vi "pathplan_vertices.vi"(0 "终点":dbl[](array[numeric]), 1 "车宽的一半":dbl=200.0, 2 "z_angle":dbl, 3 "起点":dbl[](array[numeric])) -> (7 "vertices":dbl[][](array[numeric]), 8 "distance_all":dbl, 9 "angle_all":dbl[](array[numeric]), 10 "distance_send_speed":dbl[](array[numeric]))   [LabVIEW 2016]
uses:
  <vilib>/imath/engines/lvmath2/RunTimeEngine/IndexRead/NIMS V(S).vi
  <instcachedir>/0/NIMS V(S)_0488751826AF41519A22953C041130DC.lvgen/NIMS V(S)_0488751826AF41519A22953C041130DC_000.vi
  <vilib>/imath/engines/lvmath2/RunTimeEngine/ErrorHandling/NIMS_Create Error From Enums.vi
  <vilib>/imath/engines/lvmath2/RunTimeEngine/BuiltInFunctions/length/NIMS_length(GV).vi
  <instcachedir>/0/NIMS_length(GV)_08A3D13377FD4E4B96F5795FBF3698FA.lvgen/NIMS_length(GV)_08A3D13377FD4E4B96F5795FBF3698FA_002.vi
  <vilib>/imathl/engines/lvmath/Functions/Error Handling/Create Error.vi
  <vilib>/imath/engines/lvmath/Functions/Error Handling/MergeErrorsWrapper.vi
  <vilib>/imath/engines/lvmath2/RunTimeEngine/VariableToken/NIMS_VariableToken_CondDefined.vi
  <instcachedir>/0/NIMS_VariableToken_CondDefined_06E9DA95BD4D46A6BA55EC651A891960.lvgen/NIMS_VariableToken_CondDefined_06E9DA95BD4D46A6BA55EC651A891960_003.vi
  <instcachedir>/0/NIMS_VariableToken_CondDefined_06E9DA95BD4D46A6BA55EC651A891960.lvgen/NIMS_VariableToken_CondDefined_06E9DA95BD4D46A6BA55EC651A891960_007.vi
  <vilib>/imath/engines/lvmath2/RunTimeEngine/BuiltInFunctions/size/NIMS_I32Row=size(GRow).vi
  <instcachedir>/0/NIMS_I32Row=size(GRow)_E5C05C6B13124B29B774CC4F993D3C59.lvgen/NIMS_I32Row=size(GRow)_E5C05C6B13124B29B774CC4F993D3C59_001.vi
  <vilib>/imath/engines/lvmath2/RunTimeEngine/IndexRead/NIMS M(S,S).vi
  <instcachedir>/0/NIMS M(S,S)_AC51E74150A542F7991B9634C66F3096.lvgen/NIMS M(S,S)_AC51E74150A542F7991B9634C66F3096_002.vi
  <vilib>/imath/engines/lvmath2/RunTimeEngine/IndexReplace/NIMS V(S)=S.vi
  <instcachedir>/0/NIMS V(S)=S_57E16554CB8B4B90AAB163894F717546.lvgen/NIMS V(S)=S_57E16554CB8B4B90AAB163894F717546_001.vi
  <instcachedir>/0/NIMS V(S)_0488751826AF41519A22953C041130DC.lvgen/NIMS V(S)_0488751826AF41519A22953C041130DC_003.vi
  <vilib>/imath/engines/lvmath2/RunTimeEngine/BuiltInFunctions/cos/NIMS_cos(C).vi
  <instcachedir>/0/NIMS_cos(C)_16E72F160CD540219ECD29F1B2AF26E5.lvgen/NIMS_cos(C)_16E72F160CD540219ECD29F1B2AF26E5_001.vi
  <vilib>/imath/engines/lvmath2/RunTimeEngine/BuiltInFunctions/abs/NIMS_abs(signed).vi
  <instcachedir>/0/NIMS_abs(signed)_C4FCB8E6058B49B797C7C8D53CA5F6EC.lvgen/NIMS_abs(signed)_C4FCB8E6058B49B797C7C8D53CA5F6EC_002.vi
  <vilib>/imath/engines/lvmath2/RunTimeEngine/RangeToken/NIMS_Range_R2 - Integer.vi
  <instcachedir>/0/NIMS_Range_R2 - Integer_89B873E74E6E489885E44F751DD9C6BF.lvgen/NIMS_Range_R2 - Integer_89B873E74E6E489885E44F751DD9C6BF_000.vi
  <vilib>/imath/engines/lvmath2/RunTimeEngine/CommandStatement/MC_CommandStatement_break.vi
  <instcachedir>/0/NIMS V(S)_0488751826AF41519A22953C041130DC.lvgen/NIMS V(S)_0488751826AF41519A22953C041130DC_002.vi
  <vilib>/imath/engines/lvmath2/RunTimeEngine/BuiltInFunctions/power/NIMS_power.vi
  <instcachedir>/0/NIMS_power_7E25183570944F38A5D8E4A9CE38EC54.lvgen/NIMS_power_7E25183570944F38A5D8E4A9CE38EC54_016.vi
  <instcachedir>/0/NIMS_abs(signed)_C4FCB8E6058B49B797C7C8D53CA5F6EC.lvgen/NIMS_abs(signed)_C4FCB8E6058B49B797C7C8D53CA5F6EC_000.vi
  <vilib>/imath/engines/lvmath2/RunTimeEngine/BuiltInFunctions/max/2 inputs/NIMS_max(RG,RG)-no size check.vi
  <instcachedir>/0/NIMS_max(RG,RG)-no size check_F871939977644B7683C1350DCCAD7557.lvgen/NIMS_max(RG,RG)-no size check_F871939977644B7683C1350DCCAD7557_000.vi
  <vilib>/imath/engines/lvmath2/RunTimeEngine/BuiltInFunctions/min/2 inputs/NIMS_min(RG,RG)-no size check.vi
  <instcachedir>/0/NIMS_min(RG,RG)-no size check_7F67BAB91AFC452D9517D2EA1C8F5F88.lvgen/NIMS_min(RG,RG)-no size check_7F67BAB91AFC452D9517D2EA1C8F5F88_001.vi
  <vilib>/imath/engines/lvmath2/RunTimeEngine/VariableToken/NIMS_VariableToken_CondDefinedDefinedByReplace.vi
  <instcachedir>/0/NIMS_VariableToken_CondDefinedDefinedByReplace_D162CFFC24174562A9FEA619A91E1A56.lvgen/NIMS_VariableToken_CondDefinedDefinedByReplace_D162CFFC24174562A9FEA619A91E1A56_002.vi
  <instcachedir>/0/NIMS V(S)=S_57E16554CB8B4B90AAB163894F717546.lvgen/NIMS V(S)=S_57E16554CB8B4B90AAB163894F717546_003.vi
  <vilib>/imath/engines/lvmath2/RunTimeEngine/ArithmeticOperatorToken/NIMS_ArithmeticOperator_minus.vi
  <instcachedir>/0/NIMS_ArithmeticOperator_minus_E3B65B1D26A44BB184AFDC5B3F458E3D.lvgen/NIMS_ArithmeticOperator_minus_E3B65B1D26A44BB184AFDC5B3F458E3D_003.vi
  <vilib>/imath/engines/lvmath2/RunTimeEngine/BuiltInFunctions/norm/NIMS_norm(GV,DBL).vi
  <instcachedir>/0/NIMS_norm(GV,DBL)_1268AFF3C646412B8C6EA3CE75D09042.lvgen/NIMS_norm(GV,DBL)_1268AFF3C646412B8C6EA3CE75D09042_000.vi
  <vilib>/imath/engines/lvmath2/RunTimeEngine/BuiltInFunctions/max/1 input/NIMS_max(RV).vi
  <instcachedir>/0/NIMS_max(RV)_237633DB1D604D5BA7001287DF3C7957.lvgen/NIMS_max(RV)_237633DB1D604D5BA7001287DF3C7957_002.vi
  <vilib>/imath/engines/lvmath2/RunTimeEngine/BuiltInFunctions/min/1 input/NIMS_min(RV).vi
  <instcachedir>/0/NIMS_min(RV)_EE2DD3E2888846108C5160A664B67832.lvgen/NIMS_min(RV)_EE2DD3E2888846108C5160A664B67832_002.vi
  <vilib>/imath/engines/lvmath2/RunTimeEngine/MatrixToken/NIMS_MatrixToken_RV_RV.vi
  <instcachedir>/0/NIMS_MatrixToken_RV_RV_41289AEE7DB340EFBB9CA44FA48DA89B.lvgen/NIMS_MatrixToken_RV_RV_41289AEE7DB340EFBB9CA44FA48DA89B_002.vi
  <vilib>/imath/engines/lvmath2/RunTimeEngine/MatrixToken/NIMS_MatrixToken_M_RV.vi
  <instcachedir>/0/NIMS_MatrixToken_M_RV_EE14907D4B194E829889005D2F556E9C.lvgen/NIMS_MatrixToken_M_RV_EE14907D4B194E829889005D2F556E9C_001.vi
  <vilib>/imath/engines/lvmath2/RunTimeEngine/IndexRead/NIMS V(V).vi
  <instcachedir>/0/NIMS V(V)_298D9CB7BFEB42B8BC8D9C3C28AE8C70.lvgen/NIMS V(V)_298D9CB7BFEB42B8BC8D9C3C28AE8C70_001.vi
  <vilib>/imath/engines/lvmath2/RunTimeSupport/NIMS_Get Scalar_w Error.vi
  <instcachedir>/0/NIMS_Get Scalar_w Error_59CA9FB130EE450F99234B5F2CCD930E.lvgen/NIMS_Get Scalar_w Error_59CA9FB130EE450F99234B5F2CCD930E_010.vi
  <instcachedir>/0/NIMS M(S,S)_AC51E74150A542F7991B9634C66F3096.lvgen/NIMS M(S,S)_AC51E74150A542F7991B9634C66F3096_000.vi
  <instcachedir>/0/NIMS_ArithmeticOperator_minus_E3B65B1D26A44BB184AFDC5B3F458E3D.lvgen/NIMS_ArithmeticOperator_minus_E3B65B1D26A44BB184AFDC5B3F458E3D_011.vi
  <vilib>/imath/engines/lvmath2/RunTimeEngine/IndexReplace/NIMS M($,S)=M.vi
  <instcachedir>/0/NIMS M($,S)=M_4ED09617E62F4BDFBC079C86D2836811.lvgen/NIMS M($,S)=M_4ED09617E62F4BDFBC079C86D2836811_000.vi
  <vilib>/imath/engines/lvmath2/RunTimeEngine/IndexReplace/NIMS M(S,S)=S.vi
  <instcachedir>/0/NIMS M(S,S)=S_98E40400474E4398B113AE20298B4F82.lvgen/NIMS M(S,S)=S_98E40400474E4398B113AE20298B4F82_000.vi
  <vilib>/imath/engines/lvmath2/RunTimeEngine/RowToken/NIMS_RowToken_CV_CV.vi
  <instcachedir>/0/NIMS_RowToken_CV_CV_5546A0B1CA2C4E49826F811B9C073FB0.lvgen/NIMS_RowToken_CV_CV_5546A0B1CA2C4E49826F811B9C073FB0_000.vi
  <vilib>/imath/engines/lvmath2/RunTimeEngine/IndexRead/NIMS M($,S).vi
  <instcachedir>/0/NIMS M($,S)_3E5749BBB62E49528D4765A77F1F6D98.lvgen/NIMS M($,S)_3E5749BBB62E49528D4765A77F1F6D98_002.vi
  <instcachedir>/0/NIMS_min(RG,RG)-no size check_7F67BAB91AFC452D9517D2EA1C8F5F88.lvgen/NIMS_min(RG,RG)-no size check_7F67BAB91AFC452D9517D2EA1C8F5F88_002.vi
  <instcachedir>/0/NIMS_max(RG,RG)-no size check_F871939977644B7683C1350DCCAD7557.lvgen/NIMS_max(RG,RG)-no size check_F871939977644B7683C1350DCCAD7557_001.vi
  <vilib>/imath/engines/lvmath2/RunTimeEngine/RowToken/NIMS_RowToken_M_CV.vi
  <instcachedir>/0/NIMS_RowToken_M_CV_FA79F1D1D17D44459F3ED8E09EE8B625.lvgen/NIMS_RowToken_M_CV_FA79F1D1D17D44459F3ED8E09EE8B625_000.vi
  <vilib>/imath/engines/lvmath2/RunTimeEngine/BuiltInFunctions/mirrorh/NIMS_mirrorh(GM).vi
  <instcachedir>/0/NIMS_mirrorh(GM)_A650AD0D730A4A8EBE251B4C5C7CA115.lvgen/NIMS_mirrorh(GM)_A650AD0D730A4A8EBE251B4C5C7CA115_005.vi
  <instcachedir>/0/NIMS M($,S)_3E5749BBB62E49528D4765A77F1F6D98.lvgen/NIMS M($,S)_3E5749BBB62E49528D4765A77F1F6D98_000.vi
  <vilib>/imath/engines/lvmath2/RunTimeEngine/RelationalOperatorToken/NIMS_Relational_Operator_Eq.vi
  <instcachedir>/0/NIMS_Relational_Operator_Eq_FD198F059617437A8A02361002FCA645.lvgen/NIMS_Relational_Operator_Eq_FD198F059617437A8A02361002FCA645_006.vi
  <vilib>/imath/engines/lvmath2/RunTimeEngine/IndexRead/NIMS M($,R2).vi
  <instcachedir>/0/NIMS M($,R2)_D9380E19261A4ADFB2D364AF6959C6EF.lvgen/NIMS M($,R2)_D9380E19261A4ADFB2D364AF6959C6EF_001.vi
  <vilib>/imath/engines/lvmath2/RunTimeEngine/RowToken/NIMS_RowToken_M_M.vi
  <instcachedir>/0/NIMS_RowToken_M_M_968CDE3545E74ACDAEA4B48DE01EEECA.lvgen/NIMS_RowToken_M_M_968CDE3545E74ACDAEA4B48DE01EEECA_004.vi
  <vilib>/imath/engines/lvmath2/RunTimeEngine/BuiltInFunctions/length/NIMS_length(GM).vi
  <instcachedir>/0/NIMS_length(GM)_47CEC356FCE0482D9BA47DC61C99F2C7.lvgen/NIMS_length(GM)_47CEC356FCE0482D9BA47DC61C99F2C7_000.vi
  <vilib>/imath/engines/lvmath2/RunTimeEngine/BuiltInFunctions/dot/NIMS_dot(GV,GV).vi
  <instcachedir>/0/NIMS_dot(GV,GV)_B9FAA411F4494E9B94D442721014A3FA.lvgen/NIMS_dot(GV,GV)_B9FAA411F4494E9B94D442721014A3FA_000.vi
  <vilib>/imath/engines/lvmath2/RunTimeEngine/RowToken/NIMS_RowToken_M_SorRV.vi
  <instcachedir>/0/NIMS_RowToken_M_SorRV_4D710C5E6F8040F3A39B2F03436798DB.lvgen/NIMS_RowToken_M_SorRV_4D710C5E6F8040F3A39B2F03436798DB_002.vi
  <instcachedir>/0/NIMS_abs(signed)_C4FCB8E6058B49B797C7C8D53CA5F6EC.lvgen/NIMS_abs(signed)_C4FCB8E6058B49B797C7C8D53CA5F6EC_005.vi
  <vilib>/imath/engines/lvmath2/RunTimeEngine/VariableToken/Support/NIMS_Matrix Boolean Index to I32 Index.vi
  <vilib>/imath/engines/lvmath2/RunTimeEngine/IndexReplace/NIMS M(V)=S.vi
  <instcachedir>/0/NIMS M(V)=S_F2304187E1344F60ABCBE5C5CC0920F9.lvgen/NIMS M(V)=S_F2304187E1344F60ABCBE5C5CC0920F9_000.vi
  <vilib>/imath/engines/lvmath2/RunTimeEngine/BuiltInFunctions/size/NIMS_I32=size(GM,I32).vi
  <instcachedir>/0/NIMS_I32=size(GM,I32)_122058B1B3294FAEA5DC209B92B394E4.lvgen/NIMS_I32=size(GM,I32)_122058B1B3294FAEA5DC209B92B394E4_004.vi
  <instcachedir>/0/NIMS_RowToken_M_SorRV_4D710C5E6F8040F3A39B2F03436798DB.lvgen/NIMS_RowToken_M_SorRV_4D710C5E6F8040F3A39B2F03436798DB_003.vi
  <vilib>/imath/engines/lvmath2/RunTimeEngine/IndexRead/NIMS M(S).vi
  <instcachedir>/0/NIMS M(S)_B826C018497E4940AE96BD27B540B6FB.lvgen/NIMS M(S)_B826C018497E4940AE96BD27B540B6FB_000.vi
  <vilib>/imath/engines/lvmath2/RunTimeEngine/IndexReplace/NIMS M($,S)=V.vi
  <instcachedir>/0/NIMS M($,S)=V_EEA74323A7E5479BB387BE0F93352290.lvgen/NIMS M($,S)=V_EEA74323A7E5479BB387BE0F93352290_001.vi
  <vilib>/imath/engines/lvmath2/RunTimeEngine/RowToken/NIMS_RowToken_SorRV_M.vi
  <instcachedir>/0/NIMS_RowToken_SorRV_M_1F580C56DFC142B492C663A3FF978087.lvgen/NIMS_RowToken_SorRV_M_1F580C56DFC142B492C663A3FF978087_000.vi
  <vilib>/imath/engines/lvmath2/RunTimeEngine/NodeEndStatement/NIMS_NodeEndStatement_Get Vector.vi
  <instcachedir>/0/NIMS_NodeEndStatement_Get Vector_9E4547DF38A84F62A7E036B4CE3D251C.lvgen/NIMS_NodeEndStatement_Get Vector_9E4547DF38A84F62A7E036B4CE3D251C_001.vi
  <vilib>/imath/engines/lvmath2/RunTimeEngine/NodeEndStatement/NIMS_NodeEndStatement_Output.vi
  <instcachedir>/0/NIMS_NodeEndStatement_Output_53EC0D466D134D7ABD903AC30B43404B.lvgen/NIMS_NodeEndStatement_Output_53EC0D466D134D7ABD903AC30B43404B_005.vi
  <instcachedir>/0/NIMS_NodeEndStatement_Output_53EC0D466D134D7ABD903AC30B43404B.lvgen/NIMS_NodeEndStatement_Output_53EC0D466D134D7ABD903AC30B43404B_002.vi
  <instcachedir>/0/NIMS_NodeEndStatement_Output_53EC0D466D134D7ABD903AC30B43404B.lvgen/NIMS_NodeEndStatement_Output_53EC0D466D134D7ABD903AC30B43404B_001.vi
  <vilib>/imath/engines/lvmath2/RunTimeEngine/ErrorHandling/NIMS_Finalize Error.vi
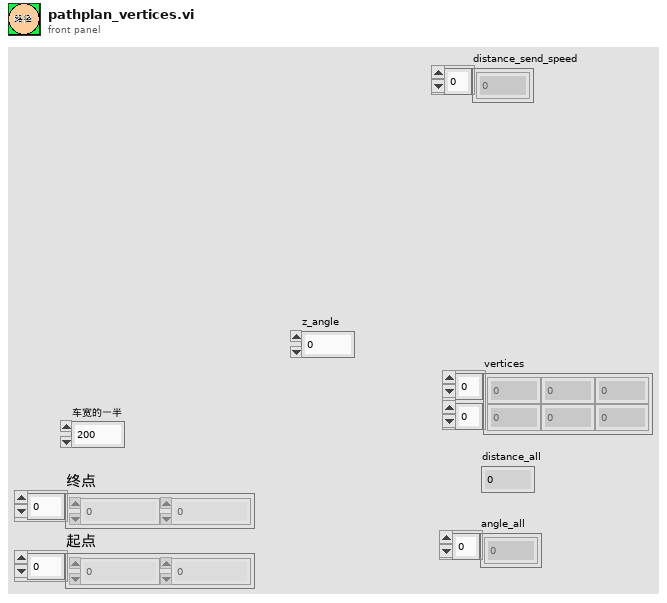
[diagram p1: front panel]
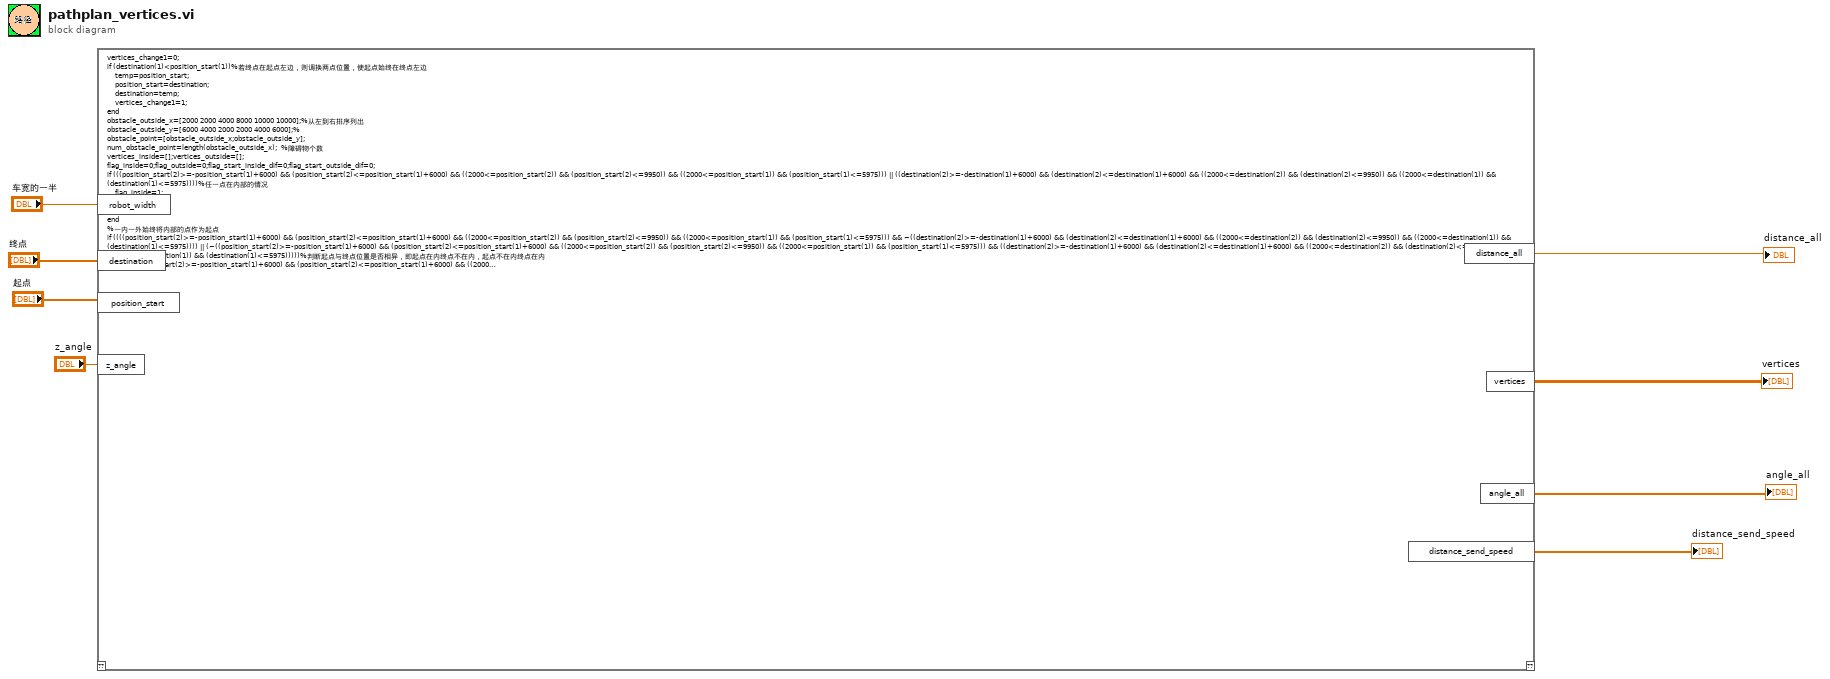
[diagram p0: block diagram]
diagram:
  n1 = mathscript code="vertices_change1=0;\nif (destination(1)<position_start(1))%若终点在起点左边，则调换两点位置，使起点始终在终点左边\n    temp=position_start;\n    position_start=destination;\n    destination=temp;\n    vertices_change1=1;\nend\nobstacle_outside_x=[2000 2000 4000 8000 10000 10000];%从左到右排序列出\nobstacle_outside_y=[6000 4000 2000 2000 4000 6000];%\nobstacle_point=[obstacle_outside_x;obstacle_outside_y];  \nnum_obstacle_point=length(obstacle_outside_x);  %障碍物个数\nvertices_inside=[];vertices_outside=[];\nflag_inside=0;flag_outside=0;flag_start_inside_dif=0;flag_start_outside_dif=0;\nif (((position_start(2)>=-position_start(1)+6000) && (position_start(2)<=position_start(1)+6000) && ((2000<=position_start(2)) && (position_start(2)<=9950)) && ((2000<=position_start(1)) && (position_start(1)<=5975))) || ((destination(2)>=-destination(1)+6000) && (destination(2)<=destination(1)+6000) && ((2000<=destination(2)) && (destination(2)<=9950)) && ((2000<=destination(1)) && (destination(1)<=5975))))%任一点在内部的情况\n    flag_inside=1;\nelse\n    flag_outside=1;\nend\n%一内一外始终将内部的点作为起点\nif ((((position_start(2)>=-position_start(1)+6000) && (position_start(2)<=position_start(1)+6000) && ((2000<=position_start(2)) && (position_start(2)<=9950)) && ((2000<=position_start(1)) && (position_start(1)<=5975))) && ~((destination(2)>=-destination(1)+6000) && (destination(2)<=destination(1)+6000) && ((2000<=destination(2)) && (destination(2)<=9950)) && ((2000<=destination(1)) && (destination(1)<=5975)))) || (~((position_start(2)>=-position_start(1)+6000) && (position_start(2)<=position_start(1)+6000) && ((2000<=position_start(2)) && (position_start(2)<=9950)) && ((2000<=position_start(1)) && (position_start(1)<=5975))) && ((destination(2)>=-destination(1)+6000) && (destination(2)<=destination(1)+6000) && ((2000<=destination(2)) && (destination(2)<=9950)) && ((2000<=destination(1)) && (destination(1)<=5975)))))%判断起点与终点位置是否相异，即起点在内终点不在内，起点不在内终点在内\n    if ((position_start(2)>=-position_start(1)+6000) && (position_start(2)<=position_start(1)+6000) && ((2000<=position_start(2)) && (position_start(2)<=9950)) && ((2000<=position_start(1)) && (position_start(1)<=5975)))%起点在内，终点在外\n        flag_start_inside_dif=1;%标记相异\n    else\n        flag_start_outside_dif=1;%标记相异，起点在外面，将点交换，内部的点作为起点\n        temp=position_start;\n        position_start=destination;\n        destination=temp;\n    end \n    position_start_inside=position_start;\n    destination_in2out=[5700 1750];%从内部到外部的目标点\nend\n\nif (flag_inside || flag_start_inside_dif || flag_start_outside_dif)%点在内部的情况\n    if (flag_start_inside_dif || flag_start_outside_dif) %如果内外相异\n        position_destination_inside=destination_in2out;\n    else   %内外不相异\n        position_start_inside=position_start;\n        position_destination_inside=destination;\n    end      \n    vertices_inside=[position_start_inside]';\n    obstacle_inside_x=[4000 6000 6000 6000];%\n    obstacle_inside_y=[6000 3500 6000 8500];%\n    size_obstacle=size(obstacle_inside_x);        %障碍物个数\n    num_obstacle=size_obstacle(1,2);\n    count=0;\n    x=[];y=[];\n    radius=150+100;\n    beta(1)=atan((position_start_inside(2)-position_destination_inside(2))/(position_start_inside(1)-position_destination_inside(1)));\n    robot_dis_obs=abs((robot_width+radius)/cos(beta(1)));\n    k=(position_start_inside(2)-position_destination_inside(2))/(position_start_inside(1)-position_destination_inside(1));\n    b=k*(-position_start_inside(1))+position_start_inside(2);\n    flag=0;\n    %判断直行路径范围内是否有障碍物，如果有记录障碍物点做标\n    if num_obstacle==0\n        x=[position_start_inside(1),position_destination_inside(1)];\n        y=[position_start_inside(2),position_destination_inside(2)];\n    else\n    for i=1:num_obstacle\n        line_k=k;line_b=b;array_o=[obstacle_inside_x(i),obstacle_inside_y(i)];\n        if line_k==inf||line_k==-inf\n            dis_dot_line=abs(array_o(2)-line_b);\n        else\n            molecule=(line_k*array_o(1)-array_o(2)+line_b);\n            dis_dot_line=abs(molecule/sqrt(power(line_k,2)+1));\n        end\n        dis_line=dis_dot_line;\n        if (dis_line<robot_width+radius || dis_line==robot_width+radius)&&(obstacle_inside_x(i)<max(position_destination_inside(1),position_start_inside(1))+robot_width+radius&&obstacle_inside_x(i)>min(position_destination_inside(1),position_start_inside(1))-robot_width+radius&&obstacle_inside_y(i)<max(position_destination_inside(2),position_start_inside(2))+robot_width+radius&&obstacle_inside_y(i)>min(position_destination_inside(2),position_start_inside(2))-robot_width+radius)\n            in_obstacle(count+1)=obstacle_inside_x(i);\n            in_obstacle(count+2)=obstacle_inside_y(i);\n            count=count+2;\n        end\n    end\n    cosalph=(position_start_inside(1)-position_destination_inside(1))/norm(position_destination_inside-position_start_inside);\n    sinalph=(position_start_inside(2)-position_destination_inside(2))/norm(position_destination_inside-position_start_inside);\n    if position_start_inside(1)<position_destination_inside(1)\n        cosalph=-cosalph;\n        sinalph=-sinalph;\n    end\n        if (count==0)       %(k==inf||k==-inf)||\n            x=[position_start_inside(1),position_destination_inside(1)];\n            y=[position_start_inside(2),position_destination_inside(2)];\n            vertices_inside=[vertices_inside,position_destination_inside'];\n        else\n            %关于障碍物点x、y轴的偏移量\n            x_offset=(robot_width+radius);\n            y_offset=(robot_width+radius);\n            %旋转坐标系下的偏移量\n            a_cos=x_offset*cosalph;a_sin=x_offset*sinalph;\n            b_cos=y_offset*cosalph;b_sin=y_offset*sinalph;\n\n            if count==2 %一个障碍物\n                %当障碍物在两点连线上方时\n                if (in_obstacle(2)>(k*in_obstacle(1)+b))||(k==inf&&position_destination_inside(1)>obstacle_inside_x(i))\n                    %先进行选取四点坐标\n                    temp_position1=[in_obstacle(1)+a_cos+b_sin,in_obstacle(2)+a_sin-b_cos];\n                    temp_position2=[in_obstacle(1)-a_cos+b_sin,in_obstacle(2)-a_sin-b_cos];\n                    if position_start_inside(1)>position_destination_inside(1)\n                        if temp_position1(1)>temp_position2(1)\n                            vertices_inside=[position_start_inside;temp_position1;temp_position2;position_destination_inside]';\n                        else\n                            vertices_inside=[position_start_inside;temp_position2;temp_position1;position_destination_inside]';\n                        end\n                    else\n                        if temp_position1(1)>temp_position2(1)\n                            vertices_inside=[position_start_inside;temp_position2;temp_position1;position_destination_inside]';\n                        else\n                            vertices_inside=[position_start_inside;temp_position1;temp_position2;position_destination_inside]';\n                        end\n                    end\n                else\n                    temp_position1=[in_obstacle(1)+a_cos-b_sin,in_obstacle(2)+a_sin+b_cos];\n                    temp_position2=[in_obstacle(1)-a_cos-b_sin,in_obstacle(2)-a_sin+b_cos];\n                    if position_start_inside(1)>position_destination_inside(1)\n                        if temp_position1(1)>temp_position2(1)\n                            vertices_inside=[position_start_inside;temp_position1;temp_position2;position_destination_inside]';\n                        else\n                            vertices_inside=[position_start_inside;temp_position2;temp_position1;position_destination_inside]';\n                        end\n                    else\n                        if temp_position1(1)>temp_position2(1)\n                            vertices_inside=[position_start_inside;temp_position2;temp_position1;position_destination_inside]';\n                        else\n                            vertices_inside=[position_start_inside;temp_position1;temp_position2;position_destination_inside]';\n                        end\n                    end\n                    for i=1:num_obstacle\n                         if (obstacle_inside_x(i)~=in_obstacle(1))&&(obstacle_inside_x(i)<max(vertices_inside(1,1),vertices_inside(1,2))&&obstacle_inside_x(i)>min(vertices_inside(1,1),vertices_inside(1,2)))&&(obstacle_inside_y(i)<((vertices_inside(2,2)-vertices_inside(2,1))/(vertices_inside(1,2)-vertices_inside(1,1))*obstacle_inside_x(i)+vertices_inside(2,2)-(vertices_inside(2,2)-vertices_inside(2,1))/(vertices_inside(1,2)-vertices_inside(1,1))*vertices_inside(1,2)+robot_dis_obs))&&(obstacle_inside_y(i)>((vertices_inside(2,2)-vertices_inside(2,1))/(vertices_inside(1,2)-vertices_inside(1,1))*obstacle_inside_x(i)+vertices_inside(2,2)-(vertices_inside(2,2)-vertices_inside(2,1))/(vertices_inside(1,2)-vertices_inside(1,1))*vertices_inside(1,2)-robot_dis_obs))||(obstacle_inside_x(i)~=in_obstacle(1))&&(obstacle_inside_x(i)<max(vertices_inside(1,3),vertices_inside(1,4))&&obstacle_inside_x(i)>min(vertices_inside(1,3),vertices_inside(1,4)))&&(obstacle_inside_y(i)<((vertices_inside(2,4)-vertices_inside(2,3))/(vertices_inside(1,4)-vertices_inside(1,3))*obstacle_inside_x(i)+vertices_inside(2,4)-(vertices_inside(2,4)-vertices_inside(2,3))/(vertices_inside(1,4)-vertices_inside(1,3))*vertices_inside(1,4)+robot_dis_obs))&&(obstacle_inside_y(i)>((vertices_inside(2,4)-vertices_inside(2,3))/(vertices_inside(1,4)-vertices_inside(1,3))*obstacle_inside_x(i)+vertices_inside(2,4)-(vertices_inside(2,4)-vertices_inside(2,3))/(vertices_inside(1,4)-vertices_inside(1,3))*vertices_inside(1,4)-robot_dis_obs))\n                            in_obstacle(count+1)=obstacle_inside_x(i);\n                            in_obstacle(count+2)=obstacle_inside_y(i);\n                            count=count+2;\n                            break;\n                        end\n                    end\n                end\n            else\n                if k*max(obstacle_inside_x)+b<min(obstacle_inside_y)\n                    temp_position1=[max(obstacle_inside_x)+x_offset,min(obstacle_inside_y)+y_offset];\n                    temp_position2=[max(obstacle_inside_x)-x_offset,min(obstacle_inside_y)+y_offset];\n                    if norm(position_start_inside-temp_position1)<norm(position_start_inside-temp_position2)\n                        temp1=temp_position1;\n                        temp2=temp_position2;\n                    else\n                        temp1=temp_position2;\n                        temp2=temp_position1;\n                    end\n                    vertices_inside=[position_start_inside;temp1;temp2;position_destination_inside]';\n                else\n                    temp_position1=[max(obstacle_inside_x)+x_offset,max(obstacle_inside_y)-y_offset];\n                    temp_position2=[max(obstacle_inside_x)-x_offset,max(obstacle_inside_y)-y_offset];\n                    if norm(position_start_inside-temp_position1)<norm(position_start_inside-temp_position2)\n                        temp1=temp_position1;\n                        temp2=temp_position2;\n                    else\n                        temp1=temp_position2;\n                        temp2=temp_position1;\n                    end\n                    vertices_inside=[position_start_inside;temp1;temp2;position_destination_inside]';\n                end\n            end\n            if count==4%两个障碍物\n                %当两个都在直线上方时\n                if (in_obstacle(2)>(k*in_obstacle(1)+b)||in_obstacle(2)==(k*in_obstacle(1)+b))&&(in_obstacle(4)>(k*in_obstacle(3)+b)||in_obstacle(4)==(k*in_obstacle(3)+b))\n                    temp_position1=[in_obstacle(1)+a_cos+b_sin,in_obstacle(2)+a_sin-b_cos];\n                    temp_position2=[in_obstacle(1)-a_cos+b_sin,in_obstacle(2)-a_sin-b_cos];\n                    temp_position3=[in_obstacle(3)+a_cos+b_sin,in_obstacle(4)+a_sin-b_cos];\n                    temp_position4=[in_obstacle(3)-a_cos+b_sin,in_obstacle(4)-a_sin-b_cos];\n                    flag=1;\n                    if norm(position_start_inside-[in_obstacle(1),in_obstacle(2)])<norm(position_start_inside-[in_obstacle(3),in_obstacle(4)])\n                        if norm(position_start_inside-temp_position1)<norm(position_start_inside-temp_position2)\n                            temp1=temp_position1;\n                            temp2=temp_position2;\n                        else\n                            temp1=temp_position2;\n                            temp2=temp_position1;\n                        end\n                        if norm(position_destination_inside-temp_position3)<norm(position_destination_inside-temp_position4)\n                            temp3=temp_position4;\n                            temp4=temp_position3;\n                        else\n                            temp3=temp_position3;\n                            temp4=temp_position4;\n                        end\n                    else\n                        if norm(position_start_inside-temp_position3)<norm(position_start_inside-temp_position4)\n                            temp1=temp_position3;\n                            temp2=temp_position4;\n                        else\n                            temp1=temp_position4;\n                            temp2=temp_position3;\n                        end\n                        if norm(position_destination_inside-temp_position1)<norm(position_destination_inside-temp_position2)\n                            temp3=temp_position2;\n                            temp4=temp_position1;\n                        else\n                            temp3=temp_position1;\n                            temp4=temp_position2;\n                        end\n                    end\n                    vertices_inside=[position_start_inside;temp1;temp4;position_destination_inside ]';\n                    %当右侧的在直线下方，左侧的在直线上方\n                elseif in_obstacle(2)<(k*in_obstacle(1)+b)&&in_obstacle(4)>(k*in_obstacle(3)+b)\n                    temp_position1=[in_obstacle(1)+a_cos-b_sin,in_obstacle(2)+a_sin+b_cos];\n                    temp_position2=[in_obstacle(1)-a_cos-b_sin,in_obstacle(2)-a_sin+b_cos];\n                    temp_position3=[in_obstacle(3)+a_cos+b_sin,in_obstacle(4)+a_sin-b_cos];\n                    temp_position4=[in_obstacle(3)-a_cos+b_sin,in_obstacle(4)-a_sin-b_cos];\n                    if norm(position_start_inside-[in_obstacle(1),in_obstacle(2)])<norm(position_start_inside-[in_obstacle(3),in_obstacle(4)])\n                        if norm(position_start_inside-temp_position1)<norm(position_start_inside-temp_position2)\n                            temp1=temp_position1;\n                            temp2=temp_position2;\n                        else\n                            temp1=temp_position2;\n                            temp2=temp_position1;\n                        end\n                        if norm(position_destination_inside-temp_position3)<norm(position_destination_inside-temp_position4)\n                            temp3=temp_position4;\n                            temp4=temp_position3;\n                        else\n                            temp3=temp_position3;\n                            temp4=temp_position4;\n                        end\n                    else\n                        if norm(position_start_inside-temp_position3)<norm(position_start_inside-temp_position4)\n                            temp1=temp_position3;\n                            temp2=temp_position4;\n                        else\n                            temp1=temp_position4;\n                            temp2=temp_position3;\n                        end\n                        if norm(position_destination_inside-temp_position1)<norm(position_destination_inside-temp_position2)\n                            temp3=temp_position2;\n                            temp4=temp_position1;\n                        else\n                            temp3=temp_position1;\n                            temp4=temp_position2;\n                        end\n                    end\n                    vertices_inside=[position_start_inside;temp1;temp2;temp3;temp4;position_destination_inside ]';\n                else%当两点都在直线下方时\n                    temp_position1=[in_obstacle(1)+a_cos-b_sin,in_obstacle(2)+a_sin+b_cos];\n                    temp_position2=[in_obstacle(1)-a_cos-b_sin,in_obstacle(2)-a_sin+b_cos];\n                    temp_position3=[in_obstacle(3)+a_cos-b_sin,in_obstacle(4)+a_sin+b_cos];\n                    temp_position4=[in_obstacle(3)-a_cos-b_sin,in_obstacle(4)-a_sin+b_cos];\n                    if norm(position_start_inside-[in_obstacle(1),in_obstacle(2)])<norm(position_start_inside-[in_obstacle(3),in_obstacle(4)])\n                        if norm(position_start_inside-temp_position1)<norm(position_start_inside-temp_position2)\n                            temp1=temp_position1;\n                            temp2=temp_position2;\n                        else\n                            temp1=temp_position2;\n                            temp2=temp_position1;\n                        end\n                        if norm(position_destination_inside-temp_position3)<norm(position_destination_inside-temp_position4)\n                            temp3=temp_position4;\n                            temp4=temp_position3;\n                        else\n                            temp3=temp_position3;\n                            temp4=temp_position4;\n                        end\n                    else\n                        if norm(position_start_inside-temp_position3)<norm(position_start_inside-temp_position4)\n                            temp1=temp_position3;\n                            temp2=temp_position4;\n                        else\n                            temp1=temp_position4;\n                            temp2=temp_position3;\n                        end\n                        if norm(position_destination_inside-temp_position1)<norm(position_destination_inside-temp_position2)\n                            temp3=temp_position2;\n                            temp4=temp_position1;\n                        else\n                            temp3=temp_position1;\n                            temp4=temp_position2;\n                        end\n                    end\n                    vertices_inside=[position_start_inside;temp1;temp4;position_destination_inside ]';\n                end\n            end\n            if count==6\n            %当三个都在直线下方时\n                temp_position1=[in_obstacle(1)+a_cos-b_sin,in_obstacle(2)+a_sin+b_cos];\n                temp_position2=[in_obstacle(1)-a_cos-b_sin,in_obstacle(2)-a_sin+b_cos];\n                temp_position3=[in_obstacle(3)+a_cos-b_sin,in_obstacle(4)+a_sin+b_cos];\n                temp_position4=[in_obstacle(3)-a_cos-b_sin,in_obstacle(4)-a_sin+b_cos];\n                temp_position5=[in_obstacle(5)+a_cos-b_sin,in_obstacle(6)+a_sin+b_cos];\n                temp_position6=[in_obstacle(5)-a_cos-b_sin,in_obstacle(6)-a_sin+b_cos];\n                vertices_inside  = [position_start_inside;temp_position5;temp_position6;temp_position3;temp_position4;temp_position1;temp_position2;position_destination_inside]';\n                if(position_start_inside(2)<in_obstacle(end))\n                    vertices_inside(:,2)=[];\n                end\n            end\n            if(position_start_inside(2)<in_obstacle(end))                   \n                vertices_inside(:,(end-2))=[];\n            end\n            vertices_inside(2,2)=vertices_inside(2,2)-1.5*radius;\n        end\n    end\nend\n\nif (flag_outside || flag_start_inside_dif || flag_start_outside_dif)%在外部运行的情况\n\n    vertices_change2=0;\n    width=[];\n    \n    if (flag_start_inside_dif || flag_start_outside_dif)%一内一外的情况\n        position_start_add=position_destination_inside;\n        position_destination_add=destination;\n    else\n        position_start_add=position_start;\n        position_destination_add=destination;\n    end\n    \n    if (position_destination_add(1)<position_start_add(1))%若终点在起点左边，则调换两点位置\n        temp=position_start_add;\n        position_start_add=position_destination_add;\n        position_destination_add=temp;\n        vertices_change2=1;\n    end\n    \n    vertices_outside=[position_start_add'];\n        \n    for i=1:num_obstacle_point-1%判断是否相交  \n        flag_intersect=0;     \n        A=position_start_add;B=position_destination_add;C=obstacle_point(:,i)';D=obstacle_point(:,i+1)';\n        AB=B-A;CD=D-C;\n        k1=AB(2)/AB(1);\n        k2=CD(2)/CD(1);\n        if(k1==inf || k1==-inf)\n            x_intersect=B(1);\n            y2=C(2)-k2*C(1);\n            y_intersect=k2*x_intersect+y2;\n        elseif(k2==inf || k2==-inf)\n            x_intersect=D(1);\n            y1=A(2)-k1*A(1);\n            y_intersect=k1*x_intersect+y1;\n        else\n            y1=A(2)-k1*A(1);\n            y2=C(2)-k2*C(1);\n            x_intersect=(y2-y1)/(k1-k2);\n            y_intersect=k1*x_intersect+y1;\n        end\n        \n        zero_set=0.01;\n        if((min(A(1),B(1))-x_intersect<=zero_set) && (x_intersect-max(A(1),B(1))<=zero_set) && (min(C(1),D(1))-x_intersect<=zero_set) && (x_intersect-max(C(1),D(1))<=zero_set) && (min(A(2),B(2))-y_intersect<=zero_set) && (y_intersect-max(A(2),B(2))<=zero_set) && (min(C(2),D(2))-y_intersect<=zero_set) && (y_intersect-max(C(2),D(2))<=zero_set))   \n            flag_intersect=1;\n        end \n        \n        if flag_intersect==1\n            if(obstacle_point(1,i+1)'<6000)\n                width=[-2*robot_width,-2*robot_width];\n            else\n                width=[2*robot_width,-2*robot_width];\n            end\n            position_start_add=obstacle_point(:,i+1)'+width;%由起点向终点走\n            vertices_outside=[vertices_outside,position_start_add'];   \n            position_start_add=obstacle_point(:,i+1)'+0.01*width;\n       end\n    end\n    \n    if (flag_start_inside_dif || flag_start_outside_dif)%一内一外的情况\n        if (destination(1)<position_destination_add(1))\n            vertices_outside=fliplr(vertices_outside);\n        else\n            vertices_outside=[vertices_outside,position_destination_add'];\n        end\n    else\n        vertices_outside=[vertices_outside,position_destination_add'];\n    end\nend\n\nif (flag_start_inside_dif || flag_start_outside_dif)%一内一外的情况\n    if(vertices_inside(:,end)==vertices_outside(:,1))\n        vertices_outside=vertices_outside(:,2:end);\n    end\nend\n\nvertices=[vertices_inside,vertices_outside];\nif (vertices_change1==1 && flag_start_outside_dif==1)\n    vertices=fliplr(vertices);\nend\nif (vertices_change1==0 && flag_start_outside_dif==1)\n    vertices=fliplr(vertices);\nend\nif (vertices_change1==1)\n    vertices=fliplr(vertices);\nend\n\n%与x轴的角度\nx_flag=[1,0];angle_all=[];\nab=x_flag;\nfor i=1:length(vertices)-1\n    b=vertices(:,i)';c=vertices(:,i+1)';\n    bc=c-b;\n    if(ab(1)*bc(2)-ab(2)*bc(1)>=0)%bc在ab的逆时针方向\n        angle_flag=1;\n    else\n        angle_flag=-1;\n    end\n    angle_flag_test=angle_flag*(acos(dot(ab,bc)/(norm(ab)*norm(bc))))*180/pi;\n    angle_all=[angle_all,angle_flag_test];\n    angle_all=real(angle_all);\nend\nangle_all(abs(angle_all)<0.1)=0;\nangle_all=angle_all+z_angle;\nangle_all=angle_all*100*3.14/180;\n\ndistance_all=0;\nfor i=1:length(vertices)-1\n    distance_all=distance_all+norm(vertices(:,i+1)-vertices(:,i));\nend\ndistance_send_speed=[];send_set=0;\nfor i=1:size(vertices,2)-1\n    send_set=send_set+norm(vertices(:,i+1)-vertices(:,i));\n    distance_send_speed=[distance_send_speed,send_set];\nend\nif (abs(vertices(1))<1 && abs(vertices(2))<1)\n    vertices(:,1)=[0,0];\nend\ndistance_send_speed=[0,distance_send_speed];"("destination"="终点", "position_start"="起点", "robot_width"="车宽的一半", "z_angle"="z_angle") -> ("vertices"=→"vertices":dbl[][], "angle_all"=→"angle_all":dbl[], "distance_all"=→"distance_all":dbl, "distance_send_speed"=→"distance_send_speed":dbl[])  [unwired: 1 in, 1 out]
